vi "WPI_JoystickGetAxis.vi"(6 "Scaler":i8=127, 10 "Axis":T1=enum."Axis 1", 11 "JoystickDevRef":T2) -> (2 "Value":dbl, 3 "JoystickDevRef":T2)   [LabVIEW 2017]
doc: "Returns the scaled value of an axis of a joystick that you specify. Use the GetRawValue VI to return raw axis information about the joystick.\n\nThis software is licensed. Open the labview\\readme\\WPI Robotics Library Open Source License.txt file for more information."
uses:
  <vilib>/Rock Robotics/WPI/Joystick/WPI_JoystickDevRef.ctl
  <vilib>/Rock Robotics/WPI/Joystick/WPI_JoystickDeviceEnum.ctl
  <vilib>/Rock Robotics/WPI/Joystick/WPI_JoystickAxis.ctl
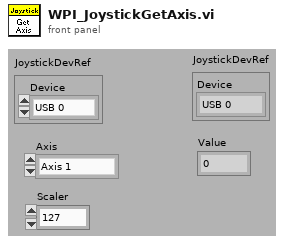
[diagram p1: front panel]
types:
  T1 = typedef "WPI_JoystickAxis.ctl" = enum16{"Axis 0", "Axis 1", "Axis 2", "Axis 3", "Axis 4", "Axis 5"}
  T2 = typedef "WPI_JoystickDevRef.ctl" = cluster{"Device":T3}
  T3 = typedef "WPI_JoystickDeviceEnum.ctl" = enum16{"USB 0", "USB 1", "USB 2", "USB 3", "USB 4", "USB 5"}
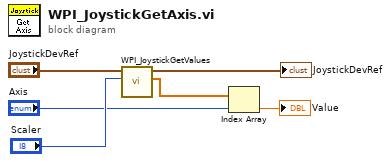
[diagram p0: block diagram]
diagram:
  n1 = call <vilib>:"WPI_JoystickGetValues.vi"("Scaler"="Scaler", "JoystickDevRef"="JoystickDevRef") -> ("Axes"=w1:dbl[], "JoystickDevRef"=→"JoystickDevRef":T2)  [unwired: 5 in, 3 out]
  n2 = Index Array(array=w1, index="Axis") -> (element=→"Value":dbl)
